vi "2D array edit.vi"(0 "min":sgl, 1 "max":sgl, 2 "Set boundaries":bool, 4 "Disabled":T1(ring), 5 "Auto close (s)":u32=120, 6 "Data Entry Limits:Increment":dbl=1.0, 7 "Display Format:Precision":u8=1, 8 "Rows":u8 min=1, 9 "Columns":u8 min=1, 10 "Caption.Text":string, 11 "Input array":sgl[][](array[numeric])=[[3.0]] caption="Y Grids" step=2) -> (3 "Output array":sgl[][](array[numeric]))   [LabVIEW 2018]
panel:
  out "Windows close (s)":u32 caption="Window closes in"
  in  "Done":bool
  # "s"
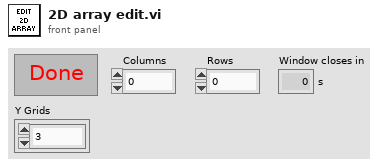
[diagram p1: front panel]
types:
  T1 = enum8{"Enabled", "Disabled", "Disabled and Grayed Out"}
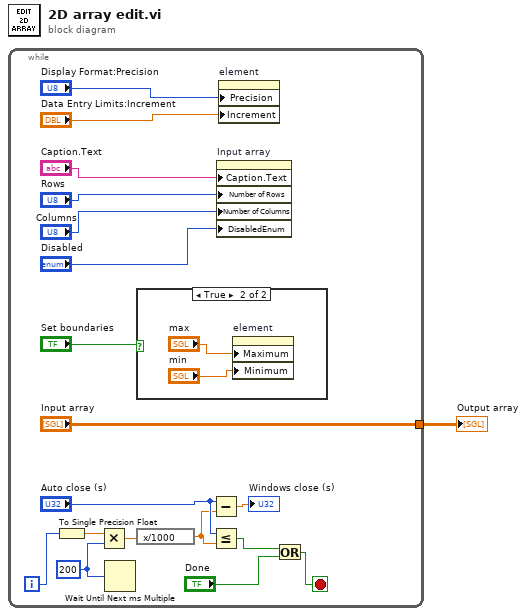
[diagram p0: block diagram]
diagram:
  n1 = while {
    tunnel: ["Input array"] -> w1
    i -> [w13]
    stop <- w11 stop-if-true
    w14 = u32 200 ("millisecond multiple")
    n2 = To Single Precision Float(number=w13) -> (single precision float=w5:sgl)
    n3 = Multiply(x=w5, y=w14) -> (x*y=w10:sgl)
    n4 = Wait Until Next ms Multiple(millisecond multiple=w14) -> ()  [unwired: 1 out]
    n5 = case shown="True" "Set boundaries" {
      frame False {
      }
      frame True {
        n6 = property on="element" class="DigNum (strict)"("Maximum"="max", "Minimum"="min") -> ()  [unwired: 2 in, 2 out]
      }
    }
    n7 = expression code="x/1000"(w10) -> (w7:sgl)
    n8 = Subtract(x="Auto close (s)", y=w7) -> (x-y=→"Windows close (s)":sgl)
    n9 = Less Or Equal?(x="Auto close (s)", y=w7) -> (x <= y?=w6:bool)
    n10 = property on="Input array" class="Arr (strict)"("Caption.Text"="Caption.Text", "Number of Rows"="Rows", "Number of Columns"="Columns", "DisabledEnum"="Disabled") -> ()  [unwired: 2 in, 2 out]
    n11 = property on="element" class="DigNum (strict)"("Precision"="Display Format:Precision", "Increment"="Data Entry Limits:Increment") -> ()  [unwired: 2 in, 2 out]
    n12 = Or(x=w6, y="Done") -> (x .or. y?=w11:bool)
  }
  "Output array" <- w1
